vi "Merge Error.vi"(10 "Error":errorcluster, 11 "Set Error in":refnum<class "jettl Event Actor.lvclass">) -> (3 "Set Error out":refnum<class "jettl Event Actor.lvclass">)   [LabVIEW 2021, in "jettl.lvlib" / "jettl Event Actor.lvlib" / "jettl Event Actor.lvclass"]
uses:
  jettl Event Actor.lvclass
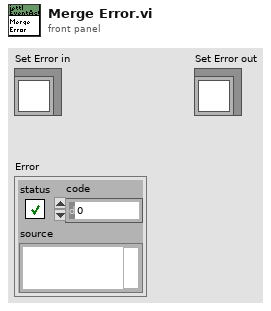
[diagram p1: front panel]
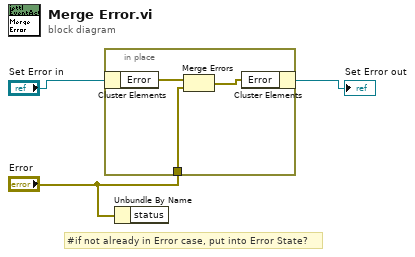
[diagram p0: block diagram]
diagram:
  # "#if not already in Error case, put into Error State?"
  n1 = in-place {
    in-place-border: "Error" -> [w4]
    n2 = in-place-cluster #1("Set Error in") -> ("Error"=w6:errorcluster)
    n3 = Merge Errors(w6, w4) -> (w5:errorcluster)
    n4 = in-place-cluster #1("Error"=w5) -> (→"Set Error out":refnum<class "jettl Event Actor.lvclass">)
  }
  n5 = Unbundle By Name("Error") -> ()  [unwired: 1 out]
